vi "Read Current Position Array.vi"(8 "error in (no error)":errorcluster, 11 "Scanner in":refnum<class "Scanner.lvclass">) -> (0 "error out":errorcluster, 2 "Position array":dbl[](array[numeric]), 3 "Scanner out":refnum<class "Scanner.lvclass">)   [LabVIEW 2012, in "Scanner.lvclass"]
uses:
  Scanner.lvclass
  Scanner.lvclass/Scanner.ctl
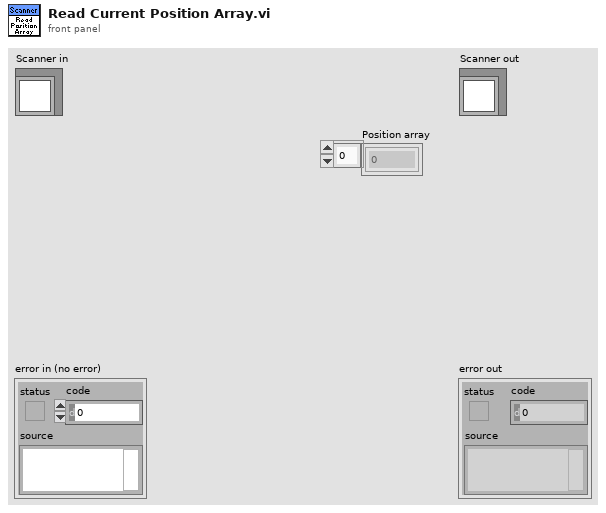
[diagram p1: front panel]
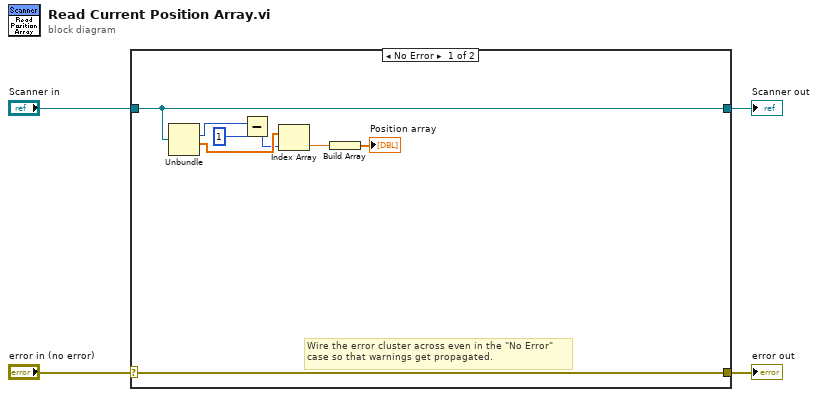
[diagram p0: block diagram]
diagram:
  n1 = case shown="No Error" "error in (no error)" {
    selector: "error in (no error)" -> [w12 w14]
    tunnel: [w12 w14] -> w3
    tunnel: [w11 w13] -> w1
    tunnel: "Scanner in" -> [w11 w13]
    frame No Error {
      # "Wire the error cluster across even in the \"No Error\"\ncase so that warnings get propagated."
      n2 = Unbundle(w11) -> (w10:u32, w8:dbl[])  [unwired: 2 out]
      n3 = Subtract(x=w10, y=u32 1) -> (x-y=w7:u32)
      n4 = Index Array(array=w8, index=w7) -> (element=w6:dbl)
      n5 = Build Array(w6) -> (→"Position array":dbl[])
    }
    frame Error {
    }
  }
  "error out" <- w3
  "Scanner out" <- w1
